vi "Merge into Object.vi"(6 "$Path or Item Name":string caption="Object $Path or Item Name", 7 "error in (no error)":errorcluster, 8 "JSON Object to Merge":string="{}", 9 "Offset":i32, 10 "JSON":string="{}") -> (0 "error out":errorcluster, 3 "<JSON>":string caption="<JSON>Merged")   [LabVIEW 2020, in "JSONtext.lvlib"]
doc: "Merges an Object into another JSON Object.\n\nMerging means that each item of the \"Object to merge\" is inserted into the other object. Insertion is at the root level unless a Path to a subObject is specified.\n\nExample: Merging {\"a\":1,\"b\":2} into {\"a\":3,\"c\":4} gives {\"a\":1,\"c\": 4,\"b\":2}\n\nNote that this merging is not recursive into subObjects."
uses:
  <vilib>/JDP Science/JSONtext/JSONtext.lvlib
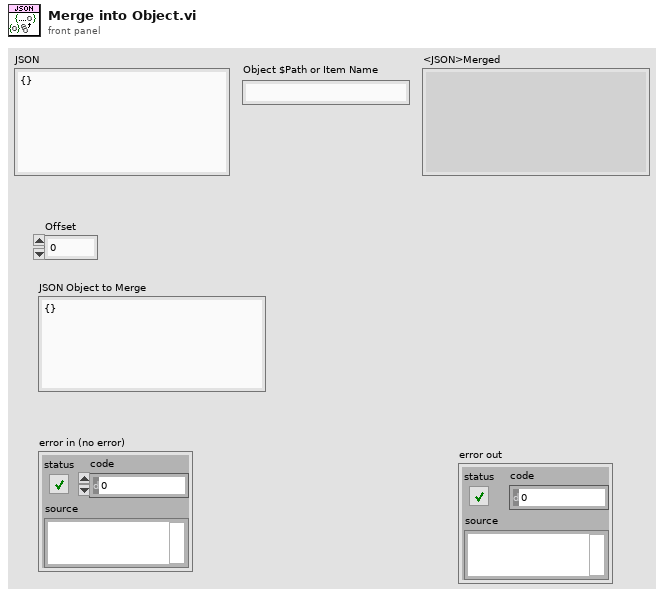
[diagram p1: front panel]
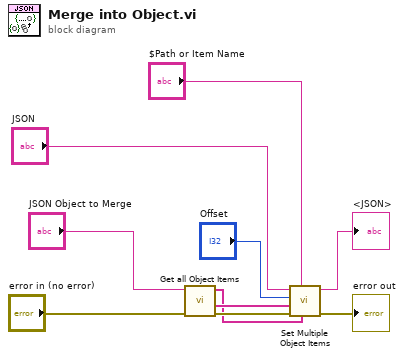
[diagram p0: block diagram]
diagram:
  n1 = call <vilib>:"Get all Object Items.vi"("error in (no error)"="error in (no error)", "JSON"="JSON Object to Merge") -> ("error out"=w10:errorcluster, "<JSON>"=w9:string[], "Item Names"=w8:string[])  [unwired: 6 in, 1 out]
  n2 = call <vilib>:"Set Multiple Object Items.vi"("Item Names"=w8, "$Path or Item Name"="$Path or Item Name", "error in (no error)"=w10, "JSON Items"=w9, "Object Offset"="Offset", "JSON"="JSON") -> ("error out"=→"error out":errorcluster, "<JSON>"=→"<JSON>":string)  [unwired: 3 in]
